vi "Write Log.vi"(8 "error in (no error)":errorcluster, 10 "Log":string, 11 "Log Folder":path) -> (0 "error out":errorcluster)   [LabVIEW 2015, in "VIDiff_Utilities.lvlib"]
uses:
  VIDiff_Utilities.lvlib
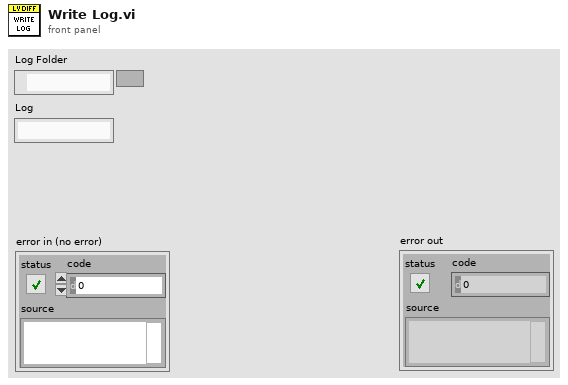
[diagram p1: front panel]
types:
  T1 = enum16{"open", "replace", "create", "open or create", "replace or create", "replace or create with confirmation"}
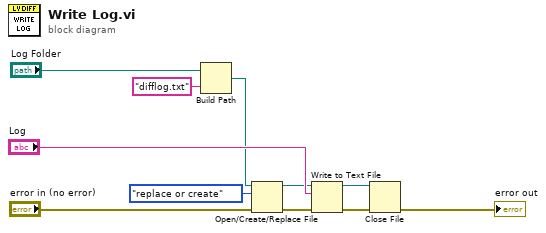
[diagram p0: block diagram]
diagram:
  n1 = Build Path(base path="Log Folder", name or relative path="difflog.txt") -> (appended path=w6:path)
  n2 = Open/Create/Replace File(file path (use dialog)=w6, error in="error in (no error)", operation (0:open)=T1."replace or create") -> (refnum out=w2:refnum<file>, error out=w5:errorcluster)  [unwired: 3 in, 1 out]
  n3 = Write to Text File(file (use dialog)=w2, text="Log", error in=w5) -> (refnum out=w3:refnum<file>, error out=w4:errorcluster)  [unwired: 1 in, 1 out]
  n4 = Close File(refnum=w3, error in=w4) -> (error out=→"error out":errorcluster)  [unwired: 1 out]
